vi "Adaptive_Indices_.vi"(2 "Patterns to Use":i32=1024, 3 "Resolution":i32=4096, 4 "Adaptive Slider":dbl(slide) scale=0.0..1.0, 5 "Compressive Indices":i32[](array[numeric])) -> (0 "Non-LUT Entries":i32[](array[numeric]), 1 "LUT":i32[](array[numeric]))   [LabVIEW 2020]
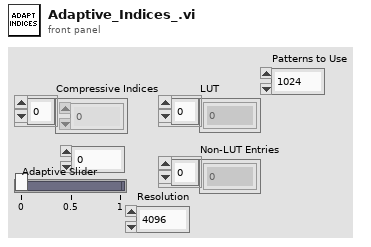
[diagram p1: front panel]
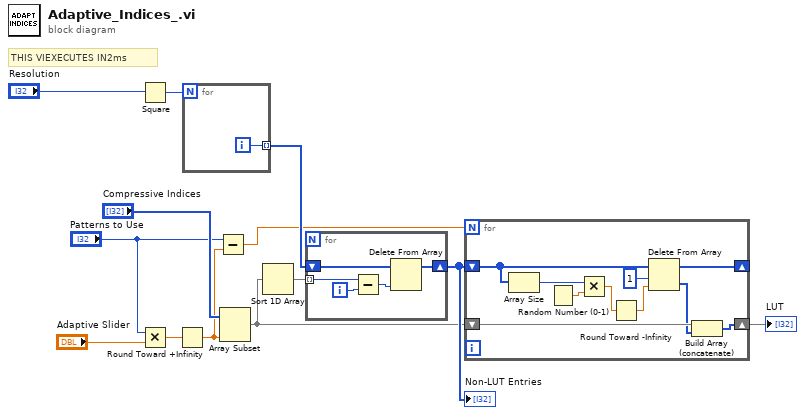
[diagram p0: block diagram]
diagram:
  # "THIS VIEXECUTES IN2ms"
  n1 = Square(x="Resolution") -> (x^2=w1:i32)
  n2 = Multiply(x="Patterns to Use", y="Adaptive Slider") -> (x*y=w5:dbl)
  n3 = Round Toward +Infinity(x=w5) -> (ceil(x): smallest int >= x=w7:dbl)
  n4 = for {
    N: w1 -> [_]
    tunnel: [w14] -> w10 mode=indexing
    i -> [w14]
  }
  n5 = Subtract(x="Patterns to Use", y=w7) -> (x-y=w6:dbl)
  n6 = Array Subset(array="Compressive Indices", length=w7) -> (w8:i32[])  [unwired: 1 in]
  n7 = Sort 1D Array(array=w8) -> (sorted array=w9:i32[])
  n8 = for {
    tunnel: w9 -> [w19] mode=indexing
    shift-right: [w15] -> w11
    shift-left: w10 -> [w17]
    i -> [w18]
    n9 = Subtract(x=w19, y=w18) -> (x-y=w16:i32)
    n10 = Delete From Array(array=w17, index=w16) -> (array with subset deleted=w15:i32[])  [unwired: 1 in, 1 out]
  }
  "Non-LUT Entries" <- w11
  n11 = for {
    N: w6 -> [_]
    shift-right: [w25] -> _
    shift-left: w11 -> [w26]
    shift-right: [w24] -> w12
    shift-left: w8 -> [w23]
    n12 = Array Size(array=w26) -> (size(s)=w28:i32)
    n13 = Random Number (0-1)() -> (number: 0 to 1=w29:dbl)
    n14 = Multiply(x=w28, y=w29) -> (x*y=w21:dbl)
    n15 = Round Toward -Infinity(1:w21) -> (0:w20:dbl)
    n16 = Delete From Array(array=w26, length=1, index=w20) -> (deleted portion=w22:i32[], array with subset deleted=w25:i32[])
    n17 = Build Array (concatenate)(w23, w22) -> (w24:i32[])
  }
  "LUT" <- w12
